vi "scan area dialog.vi"(8 "error in (no error)":errorcluster, 10 "Dongle Fitted event Refnum in":T1, 11 "Initial scanning area":T3) -> (0 "error out":errorcluster, 1 "Dongle fitted":bool, 2 "Back":bool, 3 "Scanning Area":T3)   [LabVIEW 2013]
uses:
  type_def/but_continue.ctl
  type_def/but_reload.ctl
  type_def/but_back.ctl
  type_def/Dongle fitted event refnum.ctl
  a3Di APG.lvlib
panel:
  in  "Back Button":T2
  in  "butReload":T4
  in  "Continue":T5
  in  "Scanning Area":T3 {"Scanning Area Y in mm" min=129.89 format="%#_6f"; "Scanning Area X in mm" min=184.775 format="%#_6f"}
  # "If the Panel of PCBs is on a carrier,\ndo you wish to increase the Scanning Area?\nWhen not, click Continue"
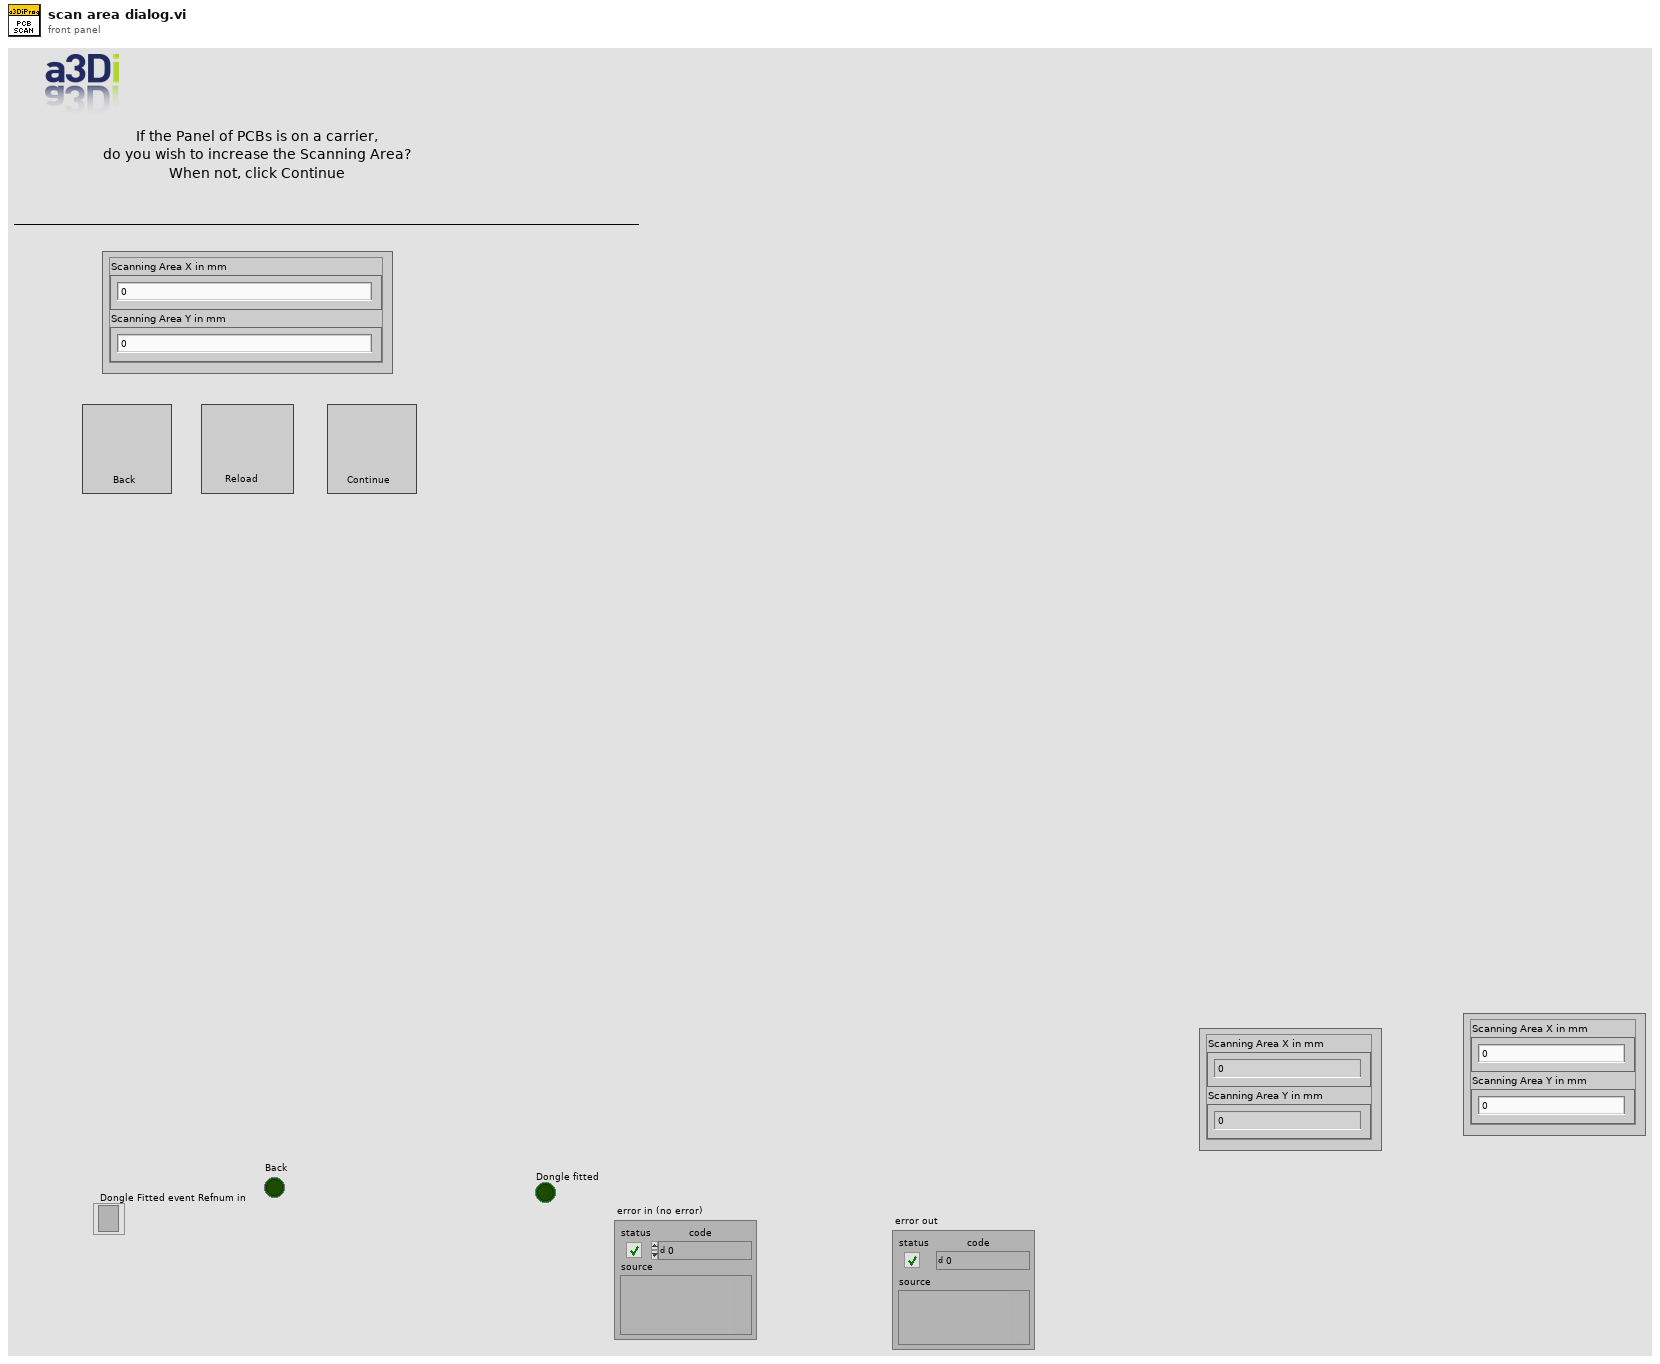
[diagram p1: front panel]
types:
  T1 = typedef "Dongle fitted event refnum.ctl" = refnum<event-registration>
  T2 = typedef "a3Di APG.lvlib/but_back.ctl" = bool
  T3 = cluster{"Scanning Area X in mm":dbl, "Scanning Area Y in mm":dbl}
  T4 = typedef "a3Di APG.lvlib/but_reload.ctl" = bool
  T5 = typedef "but_continue.ctl" = bool
  T6 = enum32{"Invalid", "Standard", "Closed", "Hidden", "Minimized", "Maximized"}
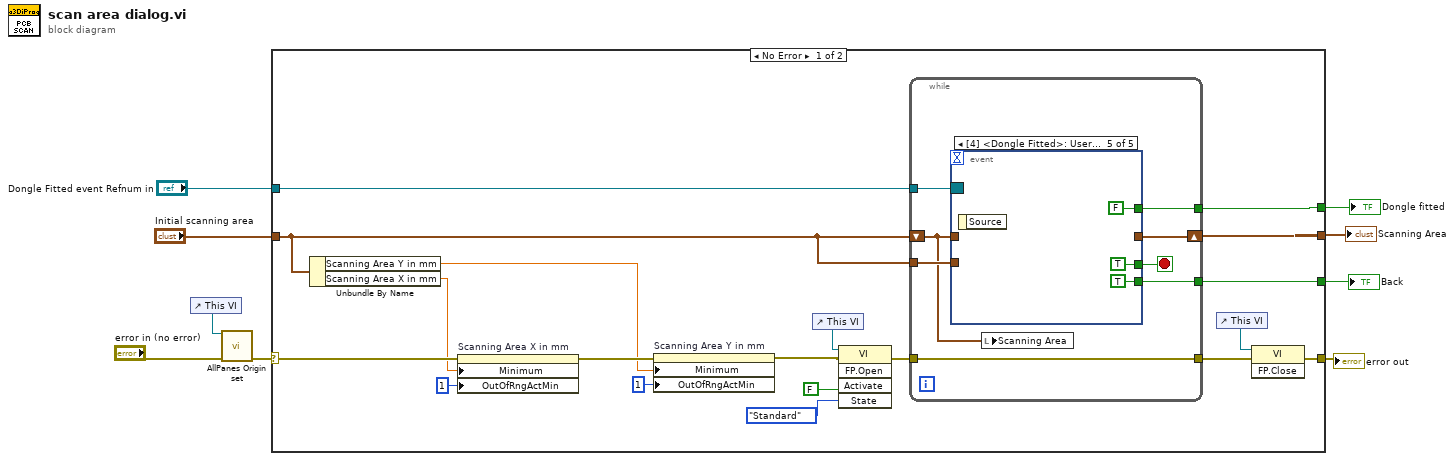
[diagram p0: block diagram]
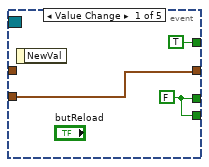
[diagram p2: hidden frame]
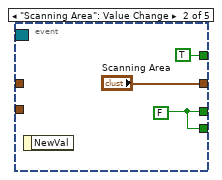
[diagram p3: hidden frame]
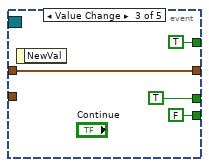
[diagram p4: hidden frame]
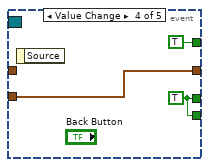
[diagram p5: hidden frame]
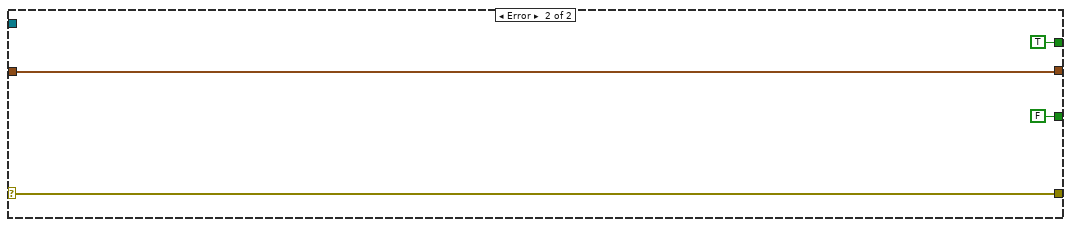
[diagram p6: hidden frame]
diagram:
  n1 = control-ref of="This VI"() -> (w4:refnum<vi>)
  n2 = call "AllPanes Origin set.vi"("VI ref in"=w4, "error in"="error in (no error)") -> ("error out"=w6:errorcluster)  [unwired: 12 in, 1 out]
  n3 = case shown="No Error" w6 {
    selector: w6 -> [w20 w56]
    tunnel: [w28 w56] -> w9
    tunnel: "Initial scanning area" -> [w15 w55]
    tunnel: [w25 w55] -> w7
    tunnel: [w12 FALSE] -> w3
    tunnel: "Dongle Fitted event Refnum in" -> [w11 _]
    tunnel: [w10 TRUE] -> w1
    frame No Error {
      n4 = Unbundle By Name(w15) -> ("Scanning Area Y in mm"=w16:dbl, "Scanning Area X in mm"=w17:dbl)
      n5 = property on="Scanning Area X in mm" class="DigNum (strict)"(error in=w20, "Minimum"=w17, "OutOfRngActMin"=u8 1 ("Response to Value Outside Limits:Minimum")) -> (error out=w19:errorcluster)  [unwired: 1 in, 1 out]
      n6 = property on="Scanning Area Y in mm" class="DigNum (strict)"(error in=w19, "Minimum"=w16, "OutOfRngActMin"=u8 1 ("Response to Value Outside Limits:Minimum")) -> (error out=w18:errorcluster)  [unwired: 1 in, 1 out]
      n7 = control-ref of="This VI"() -> (w22:refnum<vi>)
      n8 = invoke class="VI" method="FP.Open"(reference=w22, error in=w18, "Activate"=FALSE ("Activate?"), "State"=T6."Standard") -> (error out=w27:errorcluster)  [unwired: 1 in, 4 out]
      n9 = while {
        tunnel: w27 -> [w36]
        tunnel: [w36] -> w26
        shift-right: [w34] -> w25
        shift-left: w15 -> [w32]
        tunnel: w15 -> [w33]
        tunnel: [w31] -> w12
        tunnel: w11 -> [w30]
        tunnel: [w29] -> w10
        stop <- w35 stop-if-true
        n10 = event shown="[4] <Dongle Fitted>: User Event" {
          selector: w30 -> [_ _ _ _ _]
          dyn-events: _ -> [_ _ _ _ _]
          timeout: _ -> [_ _ _ _ _]
          tunnel: w32 -> [_ _ w45 _ _]
          tunnel: [w38 w41 TRUE w48 TRUE] -> w35
          tunnel: [w39 "Scanning Area" w45 w49 _] -> w34
          tunnel: w33 -> [w39 _ _ w49 _]
          tunnel: [w38 w41 FALSE w48 TRUE] -> w31
          tunnel: [TRUE TRUE TRUE TRUE FALSE] -> w29
          event Value Change {
            w38 = FALSE
            n11 = event-data() -> ()  [unwired: 1 in, 1 out]
          }
          event "Scanning Area": Value Change {
            w41 = FALSE
            n12 = event-data() -> ()  [unwired: 1 in, 1 out]
          }
          event Value Change {
            n13 = event-data() -> ()  [unwired: 1 in, 1 out]
          }
          event Value Change {
            w48 = TRUE
            n14 = event-data() -> ()  [unwired: 1 in, 1 out]
          }
          event User Event {
            n15 = event-data() -> ()  [unwired: 1 in, 1 out]
          }
        }
        n16 = local write "Scanning Area"(w32) -> ()
      }
      n17 = control-ref of="This VI"() -> (w21:refnum<vi>)
      n18 = invoke class="VI" method="FP.Close"(reference=w21, error in=w26) -> (error out=w28:errorcluster)  [unwired: 1 in, 2 out]
    }
    frame Error {
    }
  }
  "error out" <- w9
  "Scanning Area" <- w7
  "Back" <- w3
  "Dongle fitted" <- w1
